vi "Pololu-Convert Degrees Per Second to Encoder Units.vi"(4 "Degree Max":u16=180, 5 "Encoder Units Max":u16, 6 "Degree Min":u16, 7 "Encoder Units Min":u16, 8 "Error In":errorcluster, 11 "Speed (deg/sec)":u16) -> (0 "Error Out":errorcluster, 3 "Speed Encoder Units":u16)   [LabVIEW 2018]
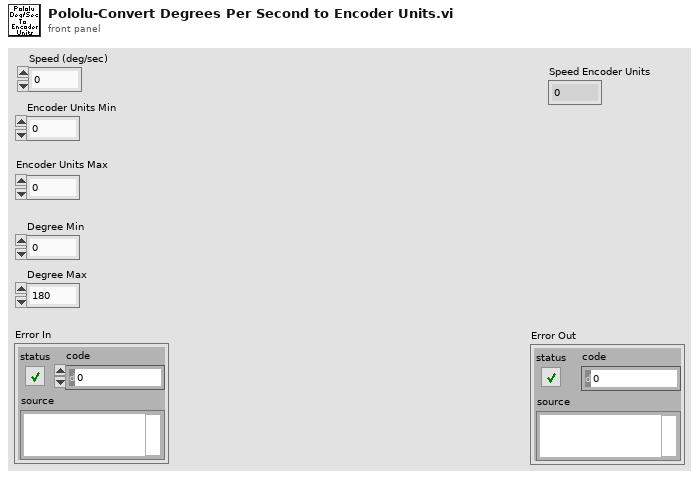
[diagram p1: front panel]
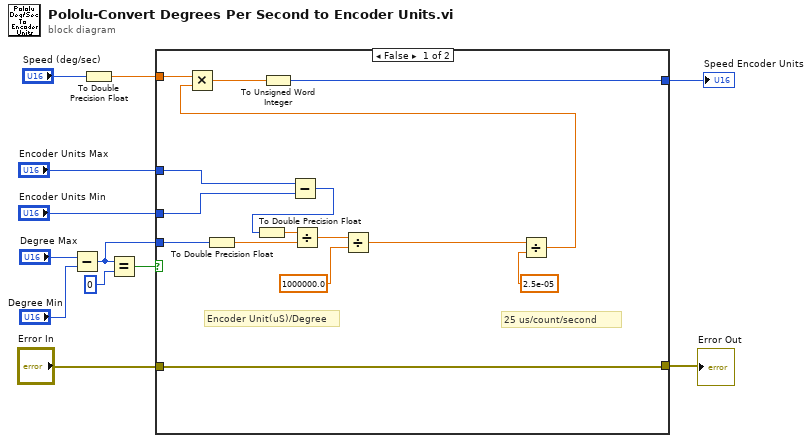
[diagram p0: block diagram]
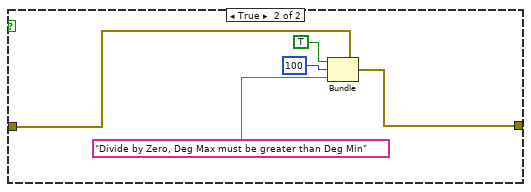
[diagram p2: hidden frame]
diagram:
  n1 = Subtract(x="Degree Max", y="Degree Min") -> (x-y=w3:u16)
  n2 = To Double Precision Float(number="Speed (deg/sec)") -> (double precision float=w12:dbl)
  n3 = Equal?(x=w3, y=u16 0) -> (x = y?=w4:bool)
  n4 = case shown="False" w4 {
    tunnel: w12 -> [w26 _]
    tunnel: "Encoder Units Max" -> [w25 _]
    tunnel: "Encoder Units Min" -> [w24 _]
    tunnel: [w18 _] -> w8
    tunnel: w3 -> [w16 _]
    tunnel: "Error In" -> [w17 w29]
    tunnel: [w17 w28] -> w1
    frame False {
      # "25 us/count/second"
      # "Encoder Unit(uS)/Degree"
      n5 = To Double Precision Float(number=w16) -> (double precision float=w15:dbl)
      n6 = Subtract(x=w25, y=w24) -> (x-y=w14:u16)
      n7 = To Double Precision Float(number=w14) -> (double precision float=w13:dbl)
      n8 = Divide(x=w13, y=w15) -> (x/y=w23:dbl)
      n9 = Divide(x=w23, y=1000000.0) -> (x/y=w21:dbl)
      n10 = Divide(x=w21, y=2.5e-05) -> (x/y=w19:dbl)
      n11 = Multiply(x=w26, y=w19) -> (x*y=w27:dbl)
      n12 = To Unsigned Word Integer(number=w27) -> (unsigned 16bit integer=w18:u16)
    }
    frame True {
      n13 = Bundle(cluster=w29, "status"=TRUE, "code"=100, "source"="Divide by Zero, Deg Max must be greater than Deg Min") -> (w28:errorcluster)
    }
  }
  "Speed Encoder Units" <- w8
  "Error Out" <- w1
